vi "CRYCheck Input Parameter.vi"(8 "Record Curve Name":string, 9 "Numeric":u16, 10 "Record Time":dbl caption="Record Time(second)" format="%#_6p", 11 "Padding Time":dbl caption="Record Padding(second)" format="%#_6p") -> (3 "Run flag":bool)   [LabVIEW 2013]
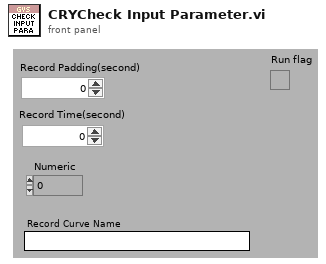
[diagram p1: front panel]
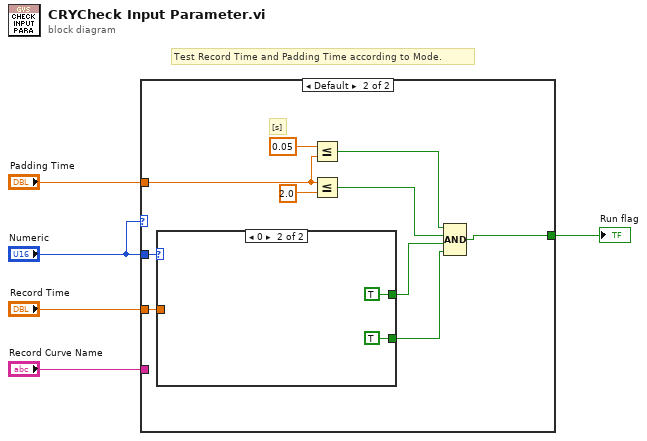
[diagram p0: block diagram]
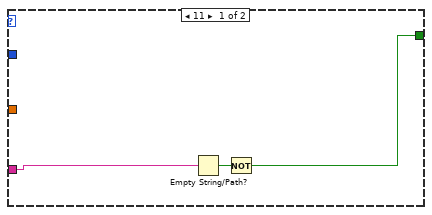
[diagram p2: hidden frame]
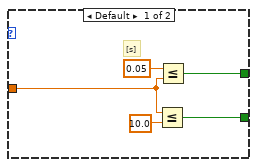
[diagram p3: hidden frame]
diagram:
  # "Test Record Time and Padding Time according to Mode."
  n1 = case shown="Default" "Numeric" {
    tunnel: "Padding Time" -> [_ w15]
    tunnel: "Record Time" -> [_ w13]
    tunnel: "Numeric" -> [_ w10]
    tunnel: [w6 w9] -> w1
    tunnel: "Record Curve Name" -> [w8 _]
    frame 11 {
      n2 = Empty String/Path?(string/path=w8) -> (empty?=w7:bool)
      n3 = Not(x=w7) -> (.not. x?=w6:bool)
    }
    frame Default {
      # "[s]"
      n4 = case shown="0" w10 {
        tunnel: w13 -> [w21 _]
        tunnel: [w20 TRUE] -> w12
        tunnel: [w19 TRUE] -> w11
        frame Default {
          # "[s]"
          n5 = Less Or Equal?(x=w21, y=10.0 ("x")) -> (x <= y?=w20:bool)
          n6 = Less Or Equal?(x=0.05, y=w21) -> (x <= y?=w19:bool)
        }
        frame 0 {
        }
      }
      n7 = Less Or Equal?(x=0.05, y=w15) -> (x <= y?=w17:bool)
      n8 = Less Or Equal?(x=w15, y=2.0 ("x")) -> (x <= y?=w14:bool)
      n9 = Compound Arithmetic op=AND(w17, w14, w11, w12) -> (w9:bool)
    }
  }
  "Run flag" <- w1
